vi "Tosca-Dirty File Check.vi"(0 "Path in":path, 1 "Action":string="continuing", 5 "Tosca":refnum<class "Parameters.lvclass">, 7 "FSM.Graph":refnum<class "FSM.Graph.lvclass">, 9 "Is Dirty?":bool, 11 "error in (no error)":errorcluster) -> (4 "Path out":path, 10 "Continue?":bool, 15 "error out":errorcluster)   [LabVIEW 2020]
uses:
  Classes/Parameters/Parameters.lvclass
  FSM Graph VIs/LV Source/Classes/FSM.Graph/FSM.Graph.lvclass
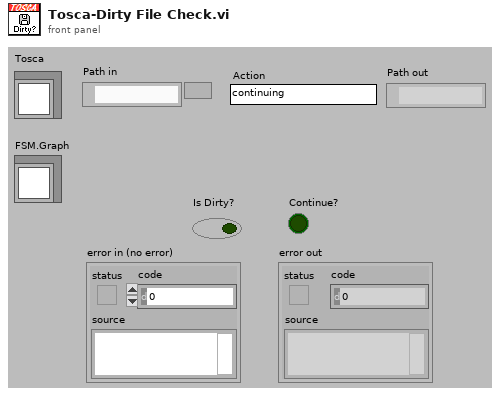
[diagram p1: front panel]
types:
  T1 = enum16{"Left Button", "Center Button", "Right Button", "Window Close"}
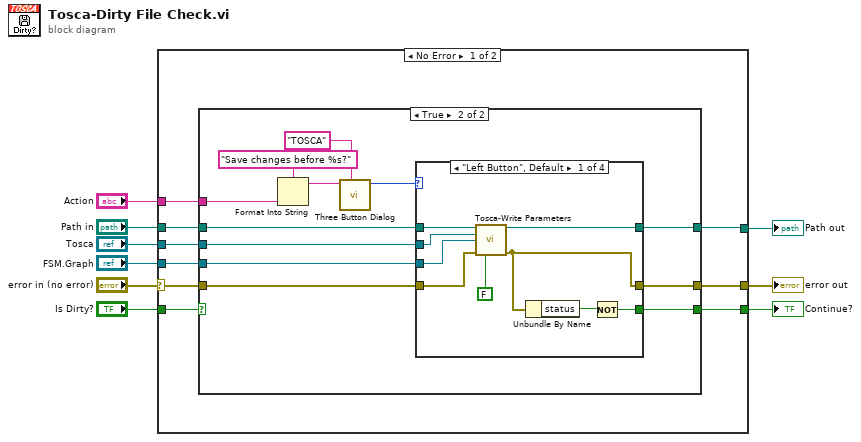
[diagram p0: block diagram]
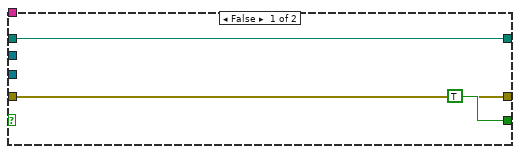
[diagram p2: hidden frame]
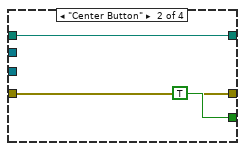
[diagram p3: hidden frame]
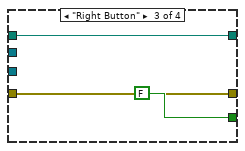
[diagram p4: hidden frame]
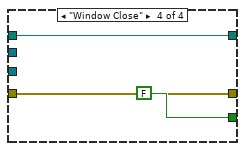
[diagram p5: hidden frame]
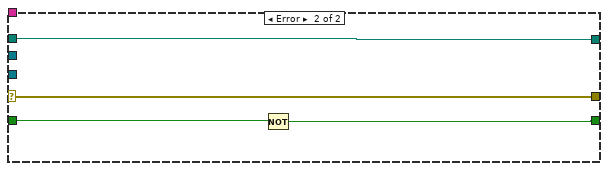
[diagram p6: hidden frame]
diagram:
  n1 = case shown="No Error" "error in (no error)" {
    selector: "error in (no error)" -> [w18 w54]
    tunnel: "Is Dirty?" -> [w17 w53]
    tunnel: "Path in" -> [w16 w55]
    tunnel: "Tosca" -> [w15 _]
    tunnel: [w14 w55] -> w5
    tunnel: "Action" -> [w13 _]
    tunnel: [w12 w52] -> w3
    tunnel: [w11 w54] -> w2
    tunnel: "FSM.Graph" -> [w10 _]
    frame No Error {
      n2 = case shown="True" w17 {
        tunnel: w18 -> [w20 w31]
        tunnel: w16 -> [w19 w33]
        tunnel: w15 -> [_ w32]
        tunnel: [w19 w30] -> w14
        tunnel: w13 -> [_ w28]
        tunnel: [TRUE w25] -> w12
        tunnel: [w20 w24] -> w11
        tunnel: w10 -> [_ w22]
        frame False {
        }
        frame True {
          n3 = Format Into String(format string="Save changes before %s?" ("message"), w28) -> (resulting string=w27:string)  [unwired: 2 in, 1 out]
          n4 = call <vilib>:"Three Button Dialog.vi"("Window Title (\"\")"="TOSCA" ("Window Title (\"\")"), "message"=w27) -> ("Which Button?"=w26:T1)  [unwired: 9 in]
          n5 = case shown="\"Left Button\", Default" w26 {
            tunnel: w33 -> [w42 w45 w47 w50]
            tunnel: w32 -> [w35 _ _ _]
            tunnel: w31 -> [w41 w43 w46 w49]
            tunnel: [w40 w45 w47 w50] -> w30
            tunnel: [w39 TRUE FALSE FALSE] -> w25
            tunnel: [w37 w43 w46 w49] -> w24
            tunnel: w22 -> [w34 _ _ _]
            frame "Left Button", Default {
              n6 = call "Tosca-Write Parameters.vi"("Path in"=w42, "Tosca"=w35, "FSM.Graph"=w34, "error in (no error)"=w41, "Prompt (T)"=FALSE) -> ("Path out"=w40:path, "error out"=w37:errorcluster)  [unwired: 8 in, 1 out]
              n7 = Unbundle By Name(w37) -> ("status"=w38:bool)
              n8 = Not(x=w38) -> (.not. x?=w39:bool)
            }
            frame "Center Button" {
            }
            frame "Right Button" {
            }
            frame "Window Close" {
            }
          }
        }
      }
    }
    frame Error {
      n9 = Not(x=w53) -> (.not. x?=w52:bool)
    }
  }
  "error out" <- w2
  "Path out" <- w5
  "Continue?" <- w3
